vi "setLevels.vi"(8 "error in (no error)":errorcluster, 10 "levels":cluster{"high":dbl, "low":dbl}, 11 "DigitalChannel.lvclass in":refnum<class "DigitalChannel.lvclass">) -> (0 "error out":errorcluster, 3 "DigitalChannel.lvclass out":refnum<class "DigitalChannel.lvclass">)   [LabVIEW 2009, in "Tools.lvlib" / "DatabaseHelpers.lvlib" / "DigitalChannel.lvclass"]
uses:
  DigitalChannel.lvclass
  DigitalChannel.lvclass/DigitalChannel.ctl
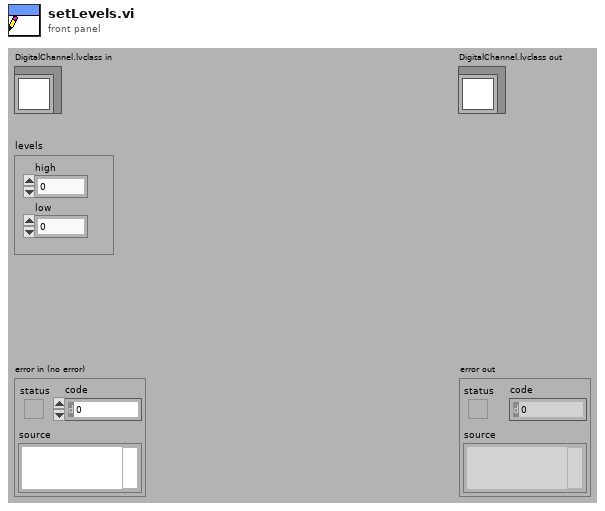
[diagram p1: front panel]
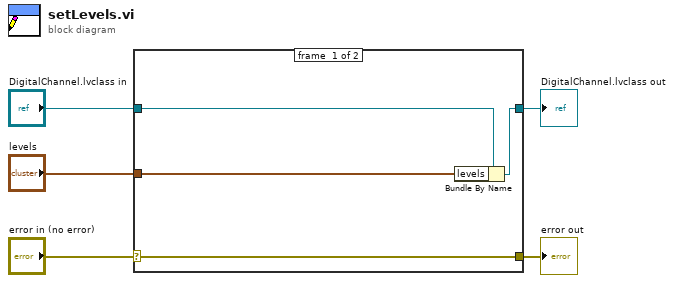
[diagram p0: block diagram]
diagram:
  n1 = case shown="No Error" "error in (no error)" {
    selector: "error in (no error)" -> [w9 w10]
    tunnel: [w9 w10] -> w4
    tunnel: [w7 w11] -> w2
    tunnel: "DigitalChannel.lvclass in" -> [w8 w11]
    tunnel: "levels" -> [w6 _]
    frame #0 {
      n2 = Bundle By Name(cluster=w8, "levels"=w6) -> (w7:refnum<class "DigitalChannel.lvclass">)
    }
    frame #1 {
    }
  }
  "error out" <- w4
  "DigitalChannel.lvclass out" <- w2
